vi "Open binary image.vi"(8 "error in":errorcluster, 11 "file path (use dialog)":path=path "\\\\vmware-host\\Shared Folders/Downloads/pug.bin") -> (0 "error out":errorcluster, 3 "data":u16[](array[numeric]) format="%.0x")   [LabVIEW 2019]
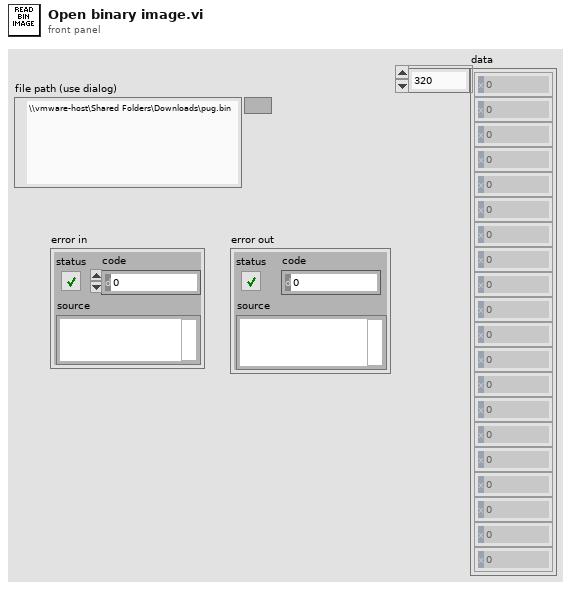
[diagram p1: front panel]
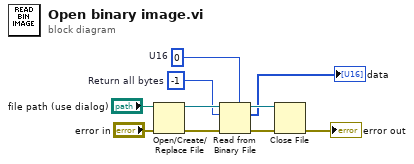
[diagram p0: block diagram]
diagram:
  w3 = u16 0  # U16
  w7 = -1  # Return all bytes
  n1 = Open/Create/Replace File(file path (use dialog)="file path (use dialog)", error in="error in") -> (refnum out=w8:refnum<file>, error out=w9:errorcluster)  [unwired: 4 in, 1 out]
  n2 = Read from Binary File(5:w3, 8:w9, 10:w7, 11:w8) -> (0:w6:errorcluster, 2:→"data":u16[], 3:w5:refnum<file>)  [unwired: 2 in, 1 out]
  n3 = Close File(refnum=w5, error in=w6) -> (error out=→"error out":errorcluster)  [unwired: 1 out]
